vi "Deadband.vi"(8 "error in (no error)":errorcluster, 11 "XBoxController in":refnum<class "XBoxController.lvclass">) -> (0 "error out":errorcluster, 3 "XBoxController out":refnum<class "XBoxController.lvclass">)   [LabVIEW 2013, in "XBoxController.lvlib" / "XBoxController.lvclass"]
uses:
  XBoxController.lvclass
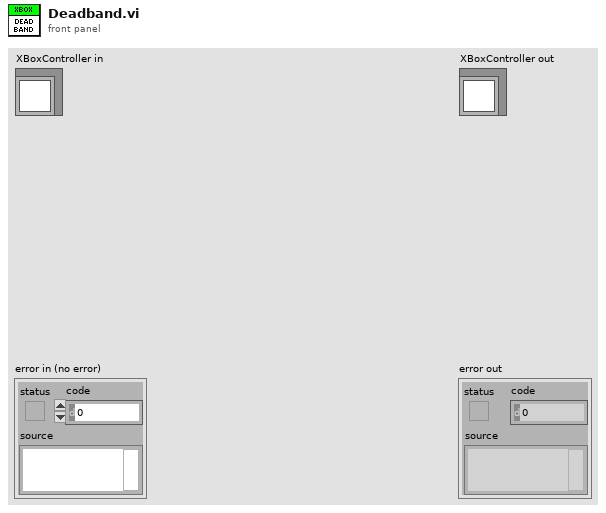
[diagram p1: front panel]
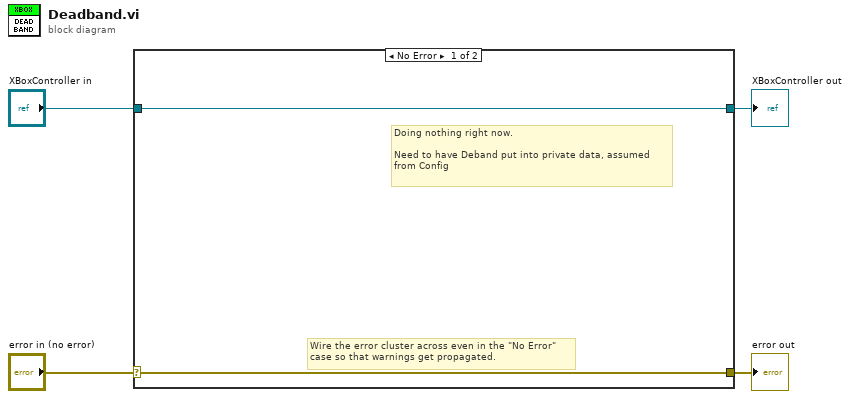
[diagram p0: block diagram]
diagram:
  n1 = case shown="No Error" "error in (no error)" {
    selector: "error in (no error)" -> [w5 w8]
    tunnel: [w5 w8] -> w3
    tunnel: [w6 w7] -> w1
    tunnel: "XBoxController in" -> [w6 w7]
    frame No Error {
      # "Doing nothing right now.\n\nNeed to have Deband put into private data, assumed\nfrom Config"
      # "Wire the error cluster across even in the \"No Error\"\ncase so that warnings get propagated."
    }
    frame Error {
    }
  }
  "error out" <- w3
  "XBoxController out" <- w1
